vi "Recognize descriptor.vi"(1 "Discriptor":dbl[](array[numeric])=[0.0, 0.0, 0.0, 0.0, 0.0, 0.0]) -> (0 "Type":enum16{"Z", "I", "O", "S", "L", "J", "T", "N"}(ring))   [LabVIEW 2018]
panel:
  out "Descriptors":dbl[][](array[numeric])
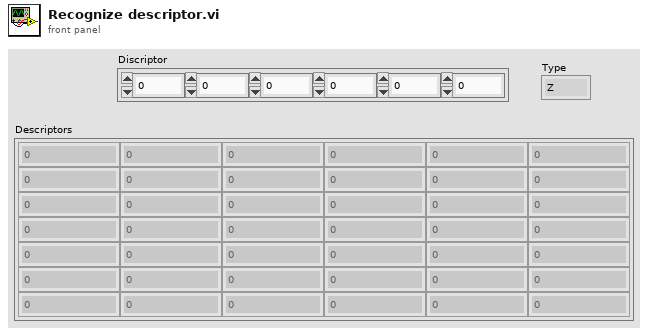
[diagram p1: front panel]
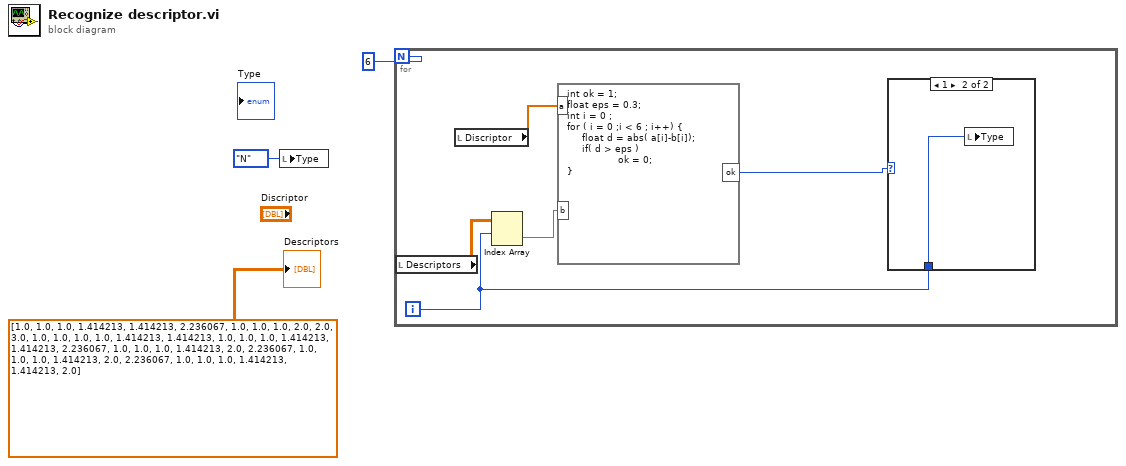
[diagram p0: block diagram]
diagram:
  n1 = local write "Type"(enum16{"Z", "I", "O", "S", "L", "J", "T", "N"}."N" ("Enum")) -> ()
  n2 = for {
    N: 6 -> [_]
    i -> [w4]
    n3 = local read "Descriptors"() -> (w8:dbl[][])
    n4 = local read "Discriptor"() -> (w7:dbl[])
    n5 = Index Array(array=w8, index (row)=w4) -> (element=w6:dbl[])  [unwired: 1 in]
    n6 = formula code="int ok = 1;\nfloat eps = 0.3;\nint i = 0 ;\nfor ( i = 0 ;i < 6 ; i++) {\n     float d = abs( a[i]-b[i]);\n     if( d > eps )\n                 ok = 0;\n}"("b"=w6, "a"=w7) -> ("ok"=w5:i32)
    n7 = case shown="1" w5 {
      tunnel: w4 -> [_ w9]
      frame 0, Default {
      }
      frame 1 {
        n8 = local write "Type"(w9) -> ()
      }
    }
  }
  "Descriptors" <- dbl[][] [[1.0, 1.0, 1.0, 1.414213, 1.414213, 2.236067], [1.0, 1.0, 1.0, 2.0, 2.0, 3.0], [1.0, 1.0, 1.0, 1.0, 1.414213, 1.414213], [1.0, 1.0, 1.0, 1.414213, 1.414213, 2.236067], [1.0, 1.0, 1.0, 1.414213, 2.0, 2.236067], [1.0, 1.0, 1.0, 1.414213, 2.0, 2.236067], [1.0, 1.0, 1.0, 1.414213, 1.414213, 2.0]] ("Descriptors")
